vi "Constructor.vi"(8 "error in (no error)":errorcluster, 11 "ScaledWaveformCalculation in":refnum<class "ScaledWaveformCalculation.lvclass">) -> (0 "error out":errorcluster, 3 "ScaledWaveformCalculation out":refnum<class "ScaledWaveformCalculation.lvclass">)   [LabVIEW 2015, in "ScaledWaveformCalculation.lvclass"]
uses:
  ScaledWaveformCalculation.lvclass
  WaveformCalculation/WaveformCalculation.lvclass/WaveformCalculation.ctl
  WaveformCalculation/WaveformCalculation.lvclass
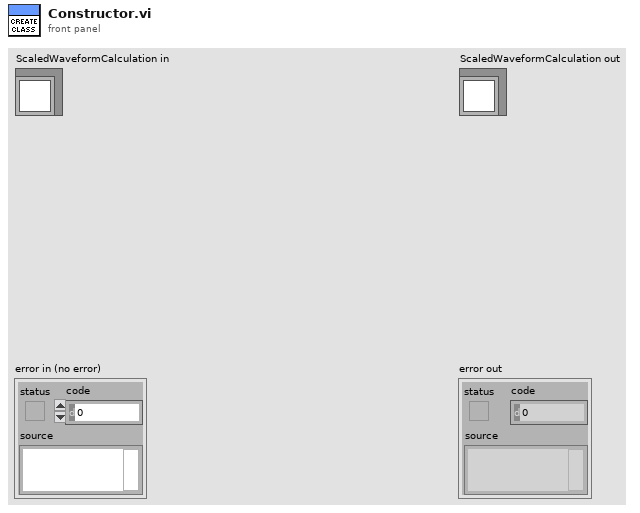
[diagram p1: front panel]
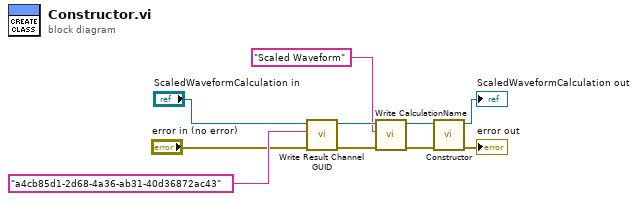
[diagram p0: block diagram]
diagram:
  n1 = call "Write Result Channel GUID.vi"("error in (no error)"="error in (no error)", "Result Channel GUID"="a4cb85d1-2d68-4a36-ab31-40d36872ac43", "WaveformCalculation in"="ScaledWaveformCalculation in") -> ("error out"=w7:errorcluster, "WaveformCalculation out"=w6:refnum<class "ScaledWaveformCalculation.lvclass">)  [unwired: 7 in]
  n2 = call "Write CalculationName.vi"("error in (no error)"=w7, "CalculationName"="Scaled Waveform", "WaveformCalculation in"=w6) -> ("error out"=w8:errorcluster, "WaveformCalculation out"=w5:refnum<class "ScaledWaveformCalculation.lvclass">)  [unwired: 7 in]
  n3 = call-parent "Constructor.vi"("error in (no error)"=w8, "WaveformCalculation in"=w5) -> ("error out"=→"error out":errorcluster, "WaveformCalculation out"=→"ScaledWaveformCalculation out":refnum<class "ScaledWaveformCalculation.lvclass">)  [unwired: 8 in]
